vi "test_libssh2_session_abstract.vi"() -> ()   [LabVIEW 2013, in "libssh2_tests.lvlib"]
uses:
  libssh2_tests.lvlib
  libssh2/libssh2_session_abstract.ctl
  libssh2/libssh2_init_default.vi
  libssh2/libssh2.lvlib
  <vilib>/addons/_JKI Toolkits/Caraya/classes/Test/Test.lvclass
  support/support.lvlib
  <vilib>/addons/_JKI Toolkits/Caraya/classes/Assert/Assert.lvclass
panel:
  out "error out":errorcluster
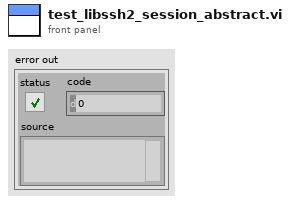
[diagram p1: front panel]
types:
  T1 = typedef "libssh2.lvlib/libssh2_session_abstract.ctl" = cluster{"send":refnum<vi>, "receive":refnum<vi>}
  T2 = typedef "libssh2.lvlib/Session Refnum.ctl" = refnum<k1>
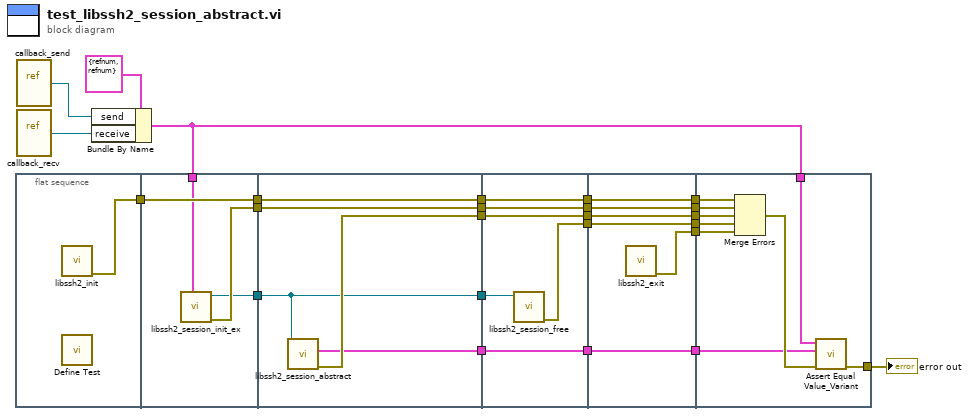
[diagram p0: block diagram]
diagram:
  n1 = flat-sequence {
    tunnel: [w26] -> w13
    tunnel: w13 -> [w30]
    tunnel: [w30] -> w11
    tunnel: [w29] -> w10
    tunnel: w1 -> [w28]
    tunnel: [w27] -> w9
    tunnel: w11 -> [w35]
    tunnel: [w35] -> w19
    tunnel: w10 -> [w34]
    tunnel: [w34] -> w18
    tunnel: [w33] -> w17
    tunnel: w9 -> [w32]
    tunnel: [w32] -> w12
    tunnel: [w31] -> w2
    tunnel: w19 -> [w41]
    tunnel: [w41] -> w8
    tunnel: w18 -> [w40]
    tunnel: [w40] -> w7
    tunnel: w17 -> [w39]
    tunnel: [w39] -> w6
    tunnel: [w38] -> w5
    tunnel: w12 -> [w37]
    tunnel: [w36] -> w3
    tunnel: w2 -> [w36]
    tunnel: w8 -> [w47]
    tunnel: [w47] -> w23
    tunnel: [w46] -> w22
    tunnel: w7 -> [w45]
    tunnel: [w45] -> w21
    tunnel: w6 -> [w44]
    tunnel: [w44] -> w20
    tunnel: [w43] -> w16
    tunnel: w5 -> [w43]
    tunnel: [w42] -> w4
    tunnel: w3 -> [w42]
    tunnel: w23 -> [w56]
    tunnel: w22 -> [w55]
    tunnel: w21 -> [w54]
    tunnel: [w52] -> w15
    tunnel: w20 -> [w51]
    tunnel: w16 -> [w50]
    tunnel: w4 -> [w49]
    tunnel: w1 -> [w48]
    frame #0 {
      n2 = call-poly "libssh2_init.vi"() -> ("error out"=w26:errorcluster)  [unwired: 11 in]
      n3 = call <vilib>:"Define Test.vi"() -> ()  [unwired: 10 in, 2 out]
    }
    frame #1 {
      n4 = call "libssh2_session_init_ex.vi"("abstract"=w28) -> ("error out"=w29:errorcluster, "session"=w27:T2)  [unwired: 9 in]
    }
    frame #2 {
      n5 = call "libssh2_session_abstract.vi"("session"=w32) -> ("error out"=w33:errorcluster, "abstract"=w31:T1)  [unwired: 9 in]
    }
    frame #3 {
      n6 = call "libssh2_session_free.vi"("session"=w37) -> ("error out"=w38:errorcluster)  [unwired: 10 in]
    }
    frame #4 {
      n7 = call "libssh2_exit.vi"() -> ("error out"=w46:errorcluster)  [unwired: 11 in]
    }
    frame #5 {
      n8 = Merge Errors(w56, w54, w51, w50, w55) -> (w53:errorcluster)
      n9 = call <vilib>:"Assert Equal Value_Variant.vi"("error in (no error)"=w53, "Y"=w49, "X"=w48) -> ("error out"=w52:errorcluster)  [unwired: 7 in, 1 out]
    }
  }
  n10 = vi-ref "callback_send.vi"() -> (w14:refnum<vi>)
  n11 = vi-ref "callback_recv.vi"() -> (w24:refnum<vi>)
  n12 = Bundle By Name(cluster=T1 {"send"=refnum, "receive"=refnum} ("abstract"), "send"=w14, "receive"=w24) -> (w1:T1)
  "error out" <- w15
